vi "QRScan_With_Manual_Input.vi"() -> ()   [LabVIEW 2016]
uses:
  <vilib>/userdefined/High Color/IMAQdx.ctl
  <vilib>/Utility/file.llb/Write Delimited Spreadsheet (string).vi
  <vilib>/vision/driver/NI_Vision_Acquisition_Software.lvlib
  <vilib>/vision/NI_Vision_Development_Module.lvlib
  <resource>/objmgr/imaqdx.rc
panel:
  out "Last Manual Input email":string
  in  "Email":string
  in  "Full Name":string
  in  "Manual":bool
  in  "file path":path
  in  "Select Resolution":u32
  out "Time":string
  out "Date":string
  out "Last Recorded Name":string
  out "Image":T1(plugin-control)
  out "Checked In":bool
  out "error out 2":errorcluster
  out "Recorded Name":string
  out "error out":errorcluster
  in  "Image Name":string="untitled"
  in  "Select Cam":T2
  in  "stop":bool
  # "Manual Check In"
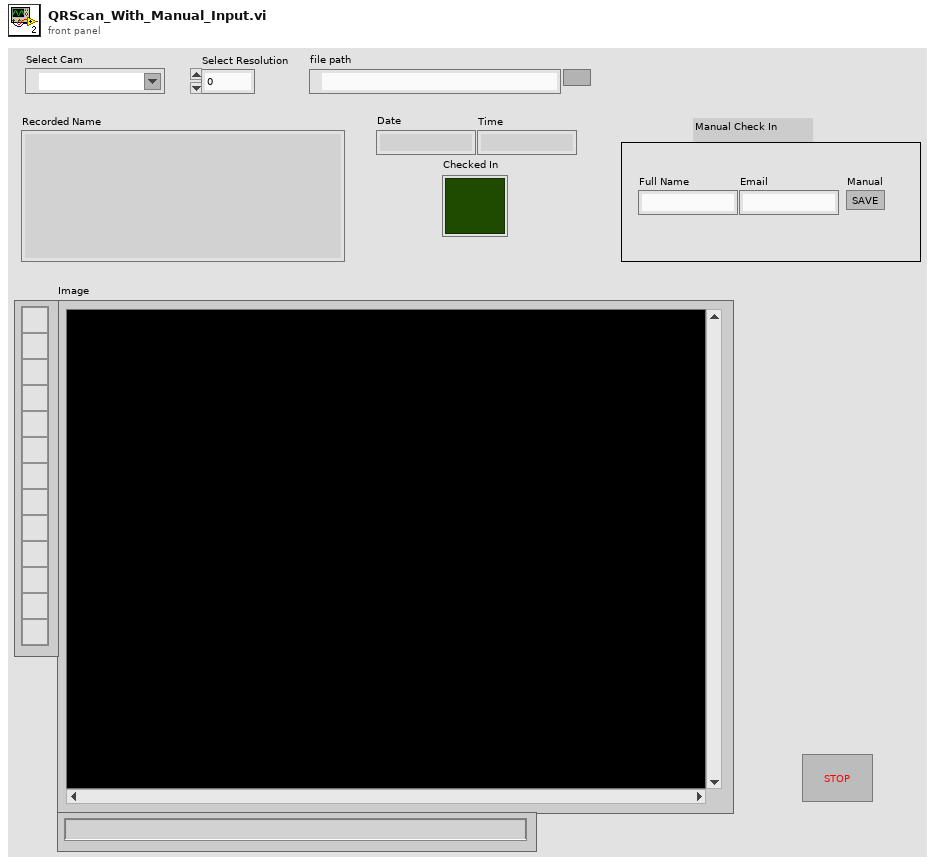
[diagram p1: front panel]
types:
  T1 = typedef "IMAQ Image.ctl" = refnum<image>
  T2 = typedef "IMAQdx.ctl" = refnum<k21>
  T3 = typedef "Image Type" = u32
  T4 = cluster{"Desired Font (Application)":enum16{"User-specified Font", "Application Font", "System Font", "Dialog Font"}, "[User-specified Font]":cluster{"Font Name":string, "Size":i16, "Strikeout?":bool, "Italic?":bool, "Underline?":bool, "Outline?":bool, "Shadow?":bool, "Bold?":bool, "Rotation Angle":dbl}, "Horizontal Alignment":i16, "Vertical Alignment":i16}
  T5 = typedef "QR Code Report.ctl" = cluster{"Found?":bool, "Data":string, "Bounding Box":cluster{"x":sgl, "y":sgl}[], "Errors Corrected":u32, "Dimensions (Rows/Cols)":u32, "Version":u32, "QR Model":T6, "Stream Mode":T7, "Barcode Polarity":T8, "Mirrored?":bool, "Append Stream Position":u32, "Size of Append Stream":u32, "First EAN-128 ID":i32, "First Alternate Language ID":i32, "Append Stream ID":u32, "Minimum Edge Strength":u32, "Demodulation Mode":T9, "Cell Sample Size":T10, "Cell Filter Mode":T11}
  T6 = typedef "QR Code Model Type.ctl" = i32
  T7 = typedef "QR Code Stream Mode Type.ctl" = i32
  T8 = typedef "Data Matrix Polarity.ctl" = i32
  T9 = typedef "Demodulation Mode.ctl" = i32
  T10 = typedef "Cell Sample Size.ctl" = i32
  T11 = typedef "Cell Filter Mode.ctl" = i32
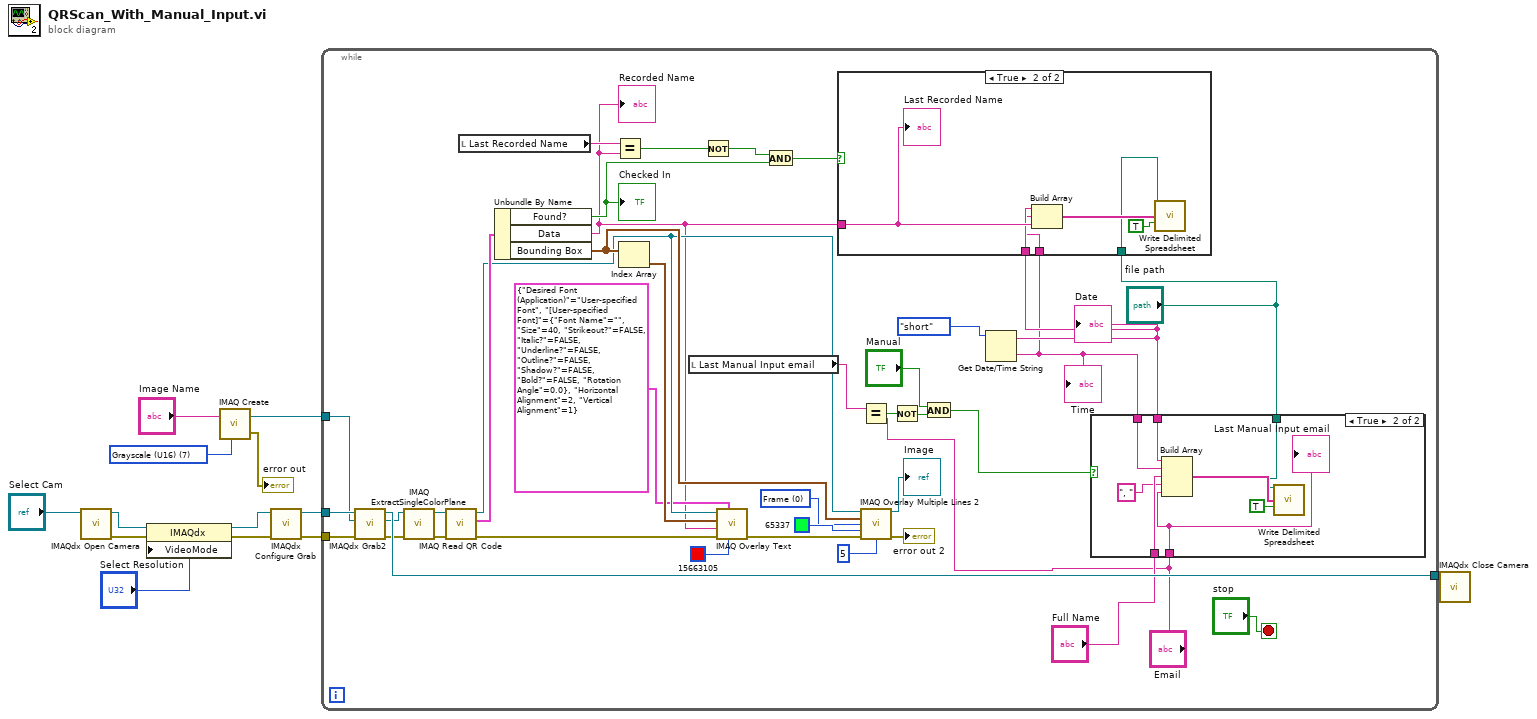
[diagram p0: block diagram]
diagram:
  w8 = T3 7 items=["Grayscale (U8)", "Grayscale (I16)", "Grayscale (SGL)", "Complex (CSG)", "RGB (U32)", "HSL (U32)", "RGB (U64)", "Grayscale (U16)"] ("Image Type")
  n1 = call <vilib>:"IMAQdx Open Camera.vi"("Session In"="Select Cam") -> ("error out"=w3:errorcluster, "Session Out"=w5:T2)  [unwired: 9 in]
  n2 = property class="IMAQdx"(reference=w5, error in=w3, "VideoMode"="Select Resolution") -> (reference out=w2:T2, error out=w4:errorcluster)
  n3 = call "IMAQ Create"("Image Name"="Image Name", "Image Type"=w8) -> ("New Image"=w7:T1, "error out"=→"error out":errorcluster)  [unwired: 3 in]
  n4 = call <vilib>:"IMAQdx Configure Grab.vi"("error in"=w4, "Session In"=w2) -> ("error out"=w10:errorcluster, "Session Out"=w11:T2)  [unwired: 8 in]
  n5 = while {
    tunnel: [w52] -> w12
    tunnel: w11 -> [w51]
    tunnel: w10 -> [w50]
    tunnel: w7 -> [w49]
    stop <- "stop" stop-if-true
    w35 = u32 0 items=["Frame", "Fill"] ("Drawing Mode (Frame)")
    n6 = call <vilib>:"IMAQdx Grab2.vi"("error in"=w50, "Image In"=w49, "Session In"=w51) -> ("error out"=w36:errorcluster, "Image Out"=w46:T1, "Session Out"=w52:T2)  [unwired: 5 in, 1 out]
    n7 = call "IMAQ ExtractSingleColorPlane"("error in (no error)"=w36, "Image Src"=w46) -> ("error out"=w47:errorcluster, "Image Dst Out"=w48:T1)  [unwired: 8 in]
    n8 = call "IMAQ Read QR Code"("error in (no error)"=w47, "Image"=w48) -> ("error out"=w38:errorcluster, "QR Code Report"=w45:T5, "Image (duplicate)"=w37:T1)  [unwired: 6 in, 1 out]
    n9 = local read "Last Recorded Name"() -> (w30:string)
    n10 = Unbundle By Name(w45) -> ("Found?"=w29:bool, "Data"=w28:string, "Bounding Box"=w42:cluster{"x":sgl, "y":sgl}[])
    "Checked In" <- w29
    "Recorded Name" <- w28
    n11 = Equal?(x=w30, y=w28) -> (x = y?=w26:bool)
    n12 = Index Array(array=w42) -> (element=w44:cluster{"x":sgl, "y":sgl})  [unwired: 1 in]
    n13 = local read "Last Manual Input email"() -> (w17:string)
    n14 = Not(x=w26) -> (.not. x?=w25:bool)
    n15 = call "IMAQ Overlay Text"("Text Color (black)"=u32 15663105, "Font, Size & Style"=T4 {"Desired Font (Application)"=enum."User-specified Font", "[User-specified Font]"={"Font Name"="", "Size"=40, "Strikeout?"=FALSE, "Italic?"=FALSE, "Underline?"=FALSE, "Outline?"=FALSE, "Shadow?"=FALSE, "Bold?"=FALSE, "Rotation Angle"=0.0}, "Horizontal Alignment"=2, "Vertical Alignment"=1}, "error in (no error)"=w38, "String"=w28, "Origin"=w44, "Image"=w37) -> ("error out"=w40:errorcluster)  [unwired: 4 in, 1 out]
    n16 = And(x=w25, y=w29) -> (x .and. y?=w27:bool)
    n17 = Equal?(x=w17, y="Email") -> (x = y?=w16:bool)
    n18 = call "IMAQ Overlay Multiple Lines 2"("Image"=w37, "Line End Points"=w42, "Drawing Mode (Frame)"=w35, "Color"=u32 65337, "error in (no error)"=w40, "Width"=u32 5) -> ("Image Out"=→"Image":T1, "error out"=→"error out 2":errorcluster)  [unwired: 8 in]
    n19 = Not(x=w16) -> (.not. x?=w15:bool)
    n20 = And(x="Manual", y=w15) -> (x .and. y?=w19:bool)
    n21 = Get Date/Time String(date format (0)=enum16{"short", "long", "abbreviated"}."short") -> (date string=w23:string, time string=w22:string)  [unwired: 2 in]
    "Date" <- w23
    "Time" <- w22
    n22 = case shown="True" w27 {
      tunnel: w28 -> [_ w64]
      tunnel: w23 -> [_ w63]
      tunnel: w22 -> [_ w62]
      tunnel: "file path" -> [_ w61]
      frame False {
      }
      frame True {
        n23 = Build Array(w63, w62, w64) -> (w65:string[])
        n24 = call-poly <vilib>:"Write Delimited Spreadsheet.vi"("file path (dialog if empty)"=w61, "1D data"=w65, "append to file? (new file:F)"=TRUE) -> ()  [unwired: 11 in, 2 out]
        "Last Recorded Name" <- w64
      }
    }
    n25 = case shown="True" w19 {
      tunnel: w23 -> [_ w60]
      tunnel: w22 -> [_ w59]
      tunnel: "file path" -> [_ w56]
      tunnel: "Email" -> [_ w53]
      tunnel: "Full Name" -> [_ w55]
      frame False {
      }
      frame True {
        n26 = Build Array(w60, w59, w55, ", " ("element"), w53) -> (w57:string[])
        n27 = call-poly <vilib>:"Write Delimited Spreadsheet.vi"("file path (dialog if empty)"=w56, "1D data"=w57, "append to file? (new file:F)"=TRUE) -> ()  [unwired: 11 in, 2 out]
        "Last Manual Input email" <- w53
      }
    }
  }
  n28 = call <vilib>:"IMAQdx Close Camera.vi"("Session In"=w12) -> ()  [unwired: 10 in, 1 out]
